vi "烧录座手动界面.vi"(8 "错误输入（无错误）":errorcluster, 10 "界面切换队列":refnum<queue>, 11 "VISA资源名称输入":refnum<visa-resource-name>) -> (0 "错误输出":errorcluster, 3 "VISA资源名称输出":refnum<visa-resource-name>)   [LabVIEW 2018]
panel:
  out "毫秒计时值":u32
  in  "枚举":T1(ring)
  in  "选项卡控件":enum32{"选项卡 1", "选项卡 2"}(tab)
  out "X30F":bool
  out "X30D":bool
  out "X30B":bool
  out "X309":bool
  out "X307":bool
  out "X305":bool
  out "X303":bool
  out "X301":bool
  out "X30E":bool
  out "X30C":bool
  out "X30A":bool
  out "X308":bool
  out "X306":bool
  out "X304":bool
  out "X302":bool
  out "写R747+读Y107+16#烧录启动":bool
  out "写R746+读Y106+14#烧录启动":bool
  out "写R745+读Y105+12#烧录启动":bool
  out "写R744+读Y104+10#烧录启动":bool
  out "写R743+读Y103+8#烧录启动":bool
  out "写R742+读Y102+6#烧录启动":bool
  out "写R741+读Y101+4#烧录启动":bool
  out "写R740+读Y100+2#烧录启动":bool
  out "写R9F+读Y30F+15#烧录启动":bool
  out "写R9E+读Y30E+13#烧录启动":bool
  out "写R9D+读Y30D+11#烧录启动":bool
  out "写R9C+读Y30C+9#烧录启动":bool
  out "写R9B+读Y30B+7#烧录启动":bool
  out "写R9A+读Y30A+5#烧录启动":bool
  out "写R99+读Y309+3#烧录启动":bool
  out "写R98+读Y308+1#烧录启动":bool
  out "写R7F+读Y307+8#烧录气缸":bool
  out "写R7E+读Y306+7#烧录气缸":bool
  out "写R7D+读Y305+6#烧录气缸":bool
  out "写R7C+读Y304+5#烧录气缸":bool
  out "写R7B+读Y303+4#烧录气缸":bool
  out "写R7A+读Y302+3#烧录气缸":bool
  out "写R79+读Y301+2#烧录气缸":bool
  out "写R78+读Y300+1#烧录气缸":bool
  out "DDT90356":dbl
  out "DDT90348":dbl
  out "自动界面":bool
  out "手动界面":bool
  out "参数界面":bool
  out "IO界面":bool
  out "产品界面":bool
  out "字符串":string
  out "DDT90352":dbl
  out "DDT90360":dbl
  out "通讯周期":dbl
  out "DT1184":T2(ring)
  out "写R0+读R1+手动启动":bool
  out "写R4+读R4+手动停止":bool
  out "写R8+读R9+机器复位":bool
  out "写R80+读R80+报警清除":bool
  out "手动5界面":bool
  out "X300":bool
  # "X"
  # "Z1"
  # "Z2"
  # "Y"
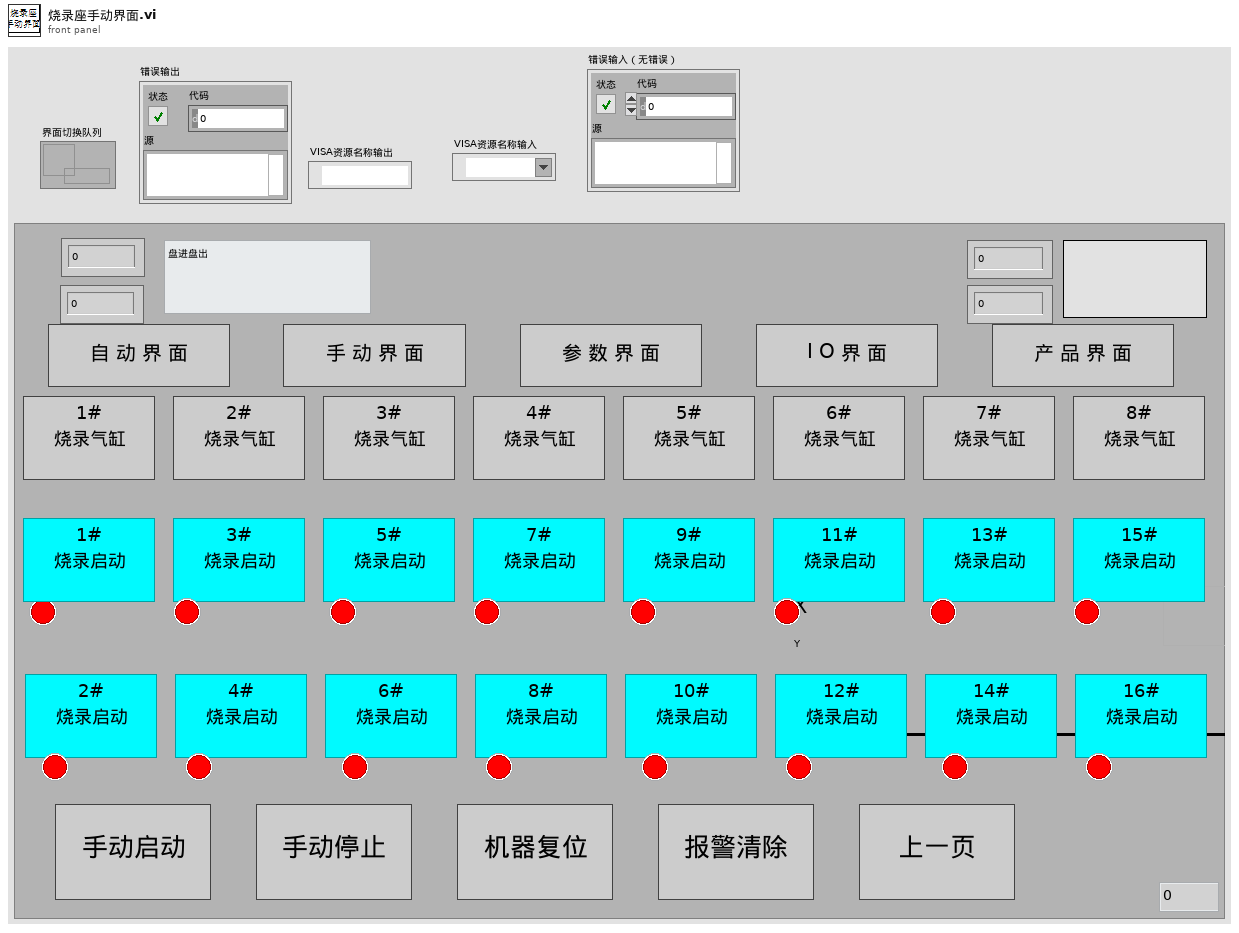
[diagram p1: front panel]
types:
  T1 = enum16{"读初始化", "读R80+8", "读R9+8", "读Y300+8", "读Y100+8", "读Y308+8", "读X308+8", "读X300+8", "读R1+8", "读DDT90356", "读DT1184", "读DDT90348", ""}
  T2 = enum16{"盘进盘出", "卷进卷出", "盘进卷出", "管进盘出", "管进卷出", "卷进盘出", ""}
  T3 = typedef "数据簇.ctl" = cluster{"字符串":string, "数值":i32, "布尔":bool}
  T4 = enum8{"Enabled", "Disabled", "Disabled and Grayed Out"}
  T5 = typedef "lveventtype.ctl" = enum32{"Null", "Timeout", "Annotation Menu Selection", "Annotation Menu Selection?", "App Instance Close", "App Instance Close?", "Autoscale Range Change", "Bookmark Info Change", "Cell Edit", "Cell Edit?", "Cursor Grab", "Cursor Grab?", "Cursor Menu Selection", "Cursor Menu Selection?", "Cursor Move", "Cursor Release", "Data Change", "Direction Change", "Display State Change", "Drag Ended", "Drag Enter", "Drag Leave", "Drag Over", "Drag Source Update", "Drag Starting", "Drag Starting?", "Drop", "Exec State Change", "Key Down", "Key Down?", "Key Repeat", "Key Repeat?", "Key Up", "Listbox Double Click", "Menu Activation?", "Menu Selection (App)", "Menu Selection? (App)", "Menu Selection (User)", "Mouse Down", "Mouse Down?", "Mouse Enter", "Mouse Leave", "Mouse Move", "Mouse Up", "Mouse Wheel", "NI Security User Change (App)", "Pane Size", "Panel Close", "Panel Close?", "Panel Resize", "Plot Attribute Change", "Scale Range Change", "Shortcut Menu Activation?", "Shortcut Menu Selection (App)", "Shortcut Menu Selection? (App)", "Shortcut Menu Selection (User)", "Tree Double Click", "Tree Drag", "Tree Drag?", "Tree Drop", "Tree Drop?", "Tree Item Close", "Tree Item Close?", "Tree Item Open", "Tree Item Open?", "User Event", "Value Change"}
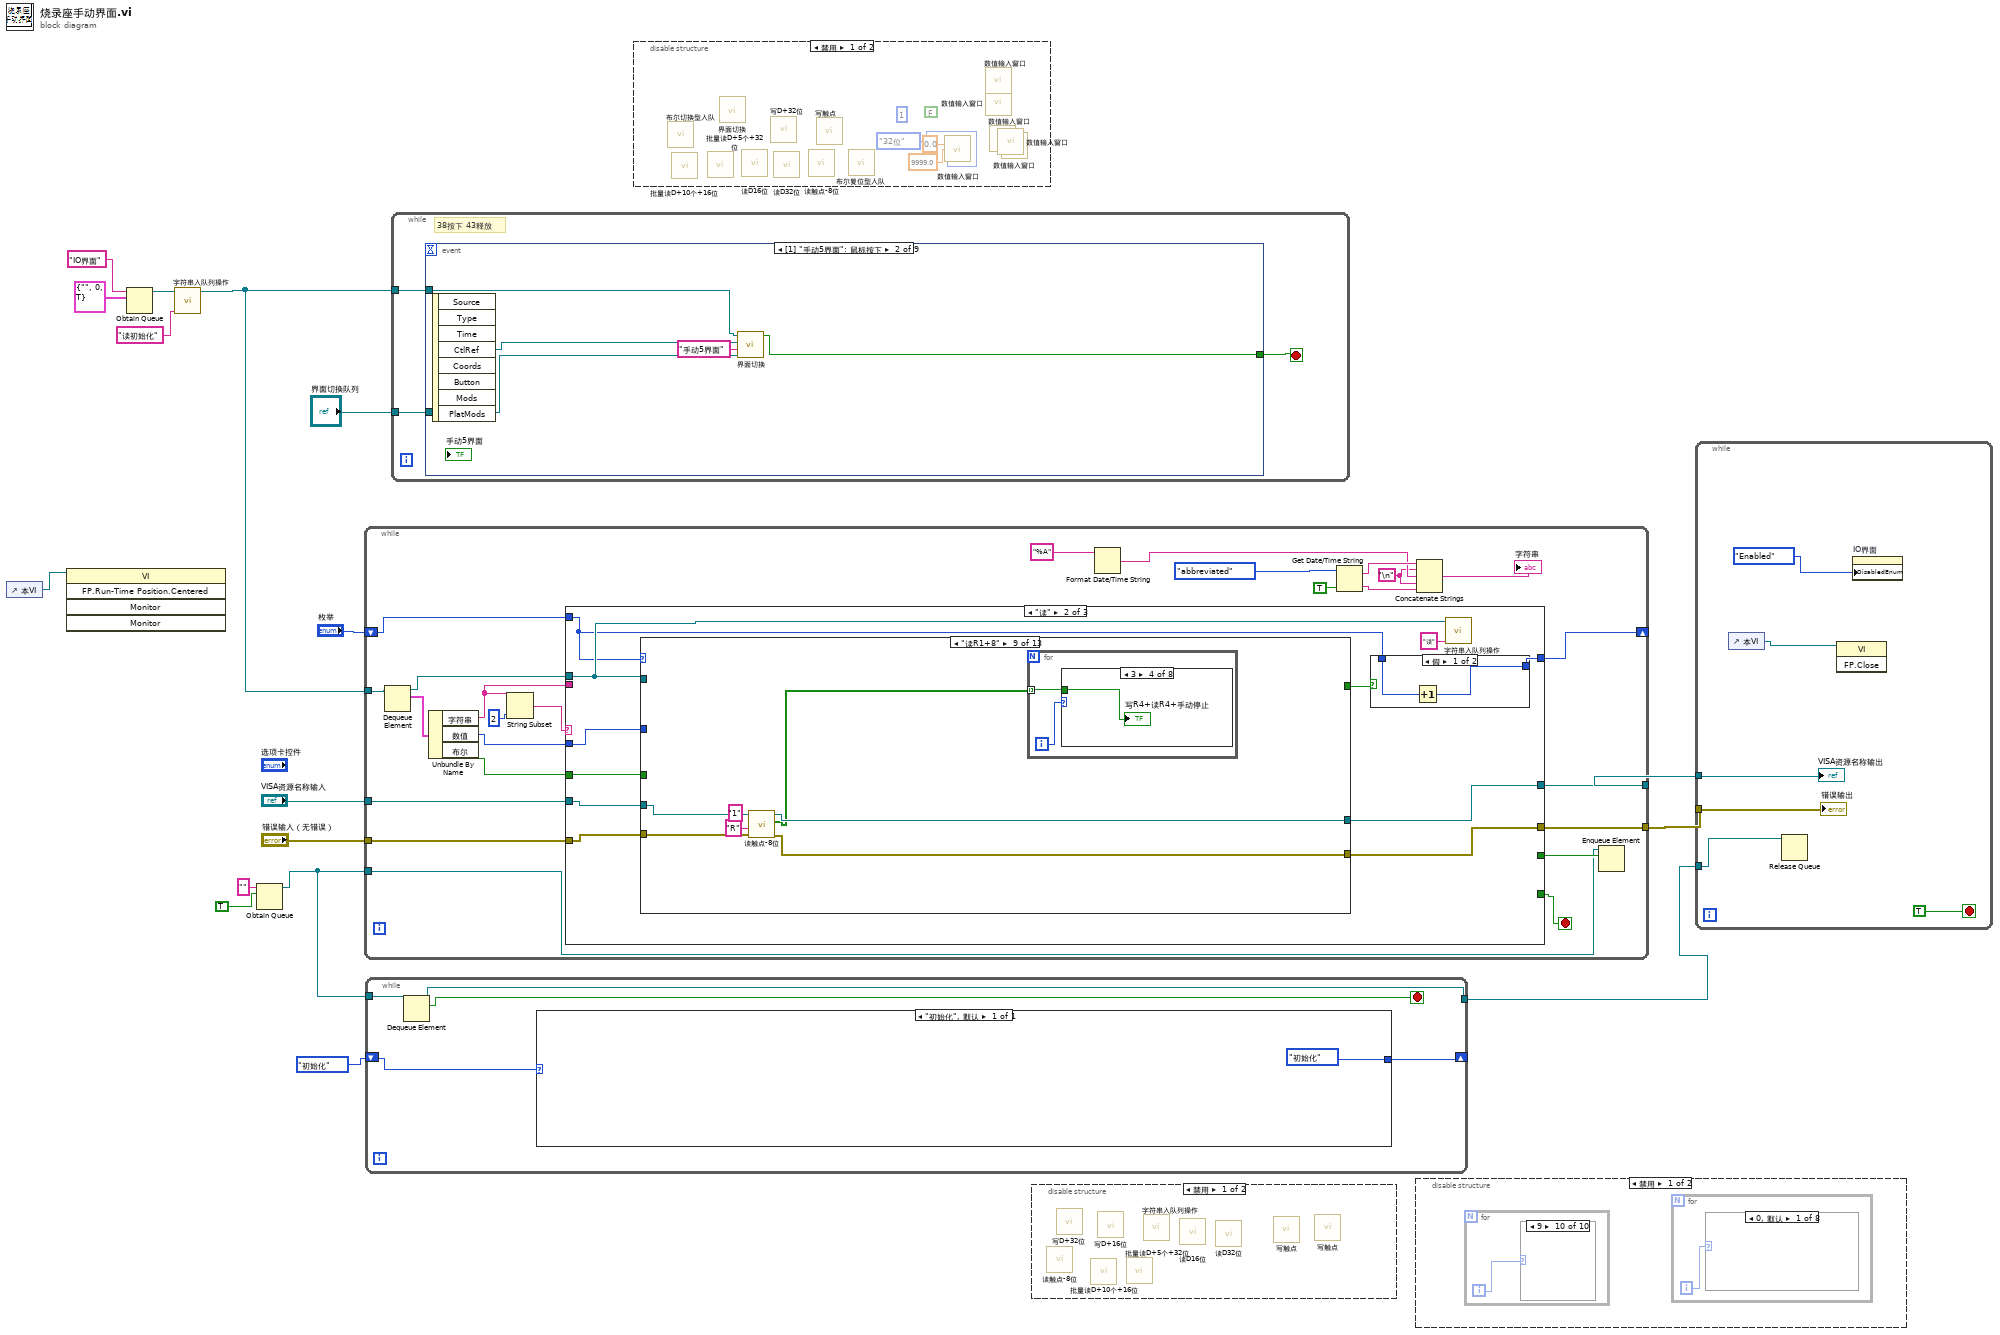
[diagram p0: block diagram]
diagram:
  n1 = control-ref of="本VI"() -> (w1:refnum<vi>)
  n2 = invoke class="VI" method="FP.Run-Time Position.Centered"(reference=w1) -> ()  [unwired: 4 in, 5 out]
  n3 = Obtain Queue(name (unnamed)="IO界面" ("名称（未命名）"), element data type=T3 {"字符串"="", "数值"=0, "布尔"=TRUE}) -> (queue out=w10:refnum<queue>)  [unwired: 3 in, 2 out]
  n4 = call "字符串入队列操作.vi"("字符消息入队列"="读初始化", "界面切换队列"=w10) -> ("队列输出"=w2:refnum<queue>)  [unwired: 9 in]
  n5 = Obtain Queue(name (unnamed)="" ("名称（未命名）"), element data type=TRUE) -> (queue out=w5:refnum<queue>)  [unwired: 3 in, 2 out]
  n6 = while {
    tunnel: w2 -> [w38]
    tunnel: "VISA资源名称输入" -> [w31]
    tunnel: "错误输入（无错误）" -> [w30]
    tunnel: [w29] -> w12
    tunnel: [w28] -> w11
    shift-right: [w25] -> _
    shift-left: "枚举" -> [w26]
    tunnel: w5 -> [w18]
    stop <- w20 stop-if-true
    w22 = "\n"
    n7 = Dequeue Element(queue=w38) -> (queue out=w35:refnum<queue>, element=w37:T3)  [unwired: 2 in, 2 out]
    n8 = Unbundle By Name(w37) -> ("字符串"=w32:string, "数值"=w34:i32, "布尔"=w33:bool)
    n9 = String Subset(string=w32, length (rest)=2 ("长度（剩余）")) -> (substring=w36:string)  [unwired: 1 in]
    n10 = case shown="\"读\"" w36 {
      selector: w36 -> [w45 _ _]
      tunnel: w35 -> [_ w53 w238]
      tunnel: w34 -> [_ w60 w237]
      tunnel: w33 -> [_ w59 w236]
      tunnel: w32 -> [_ _ w230]
      tunnel: w31 -> [w44 w58 w235]
      tunnel: w30 -> [w43 w57 w234]
      tunnel: [w44 w56 w232] -> w29
      tunnel: [w43 w55 w231] -> w28
      tunnel: [_ _ w233] -> w20
      tunnel: w26 -> [_ w51 _]
      tunnel: [_ w50 _] -> w25
      tunnel: [_ _ w228] -> w19
      frame "", Default {
        n11 = Concatenate Strings("无对应消息分支**" ("消息"), w45, "**" ("字符串"), "读写状态机" ("字符串")) -> (w47:string)
        n12 = One Button Dialog(message=w47) -> ()  [unwired: 1 in, 1 out]
      }
      frame "读" {
        n13 = case shown="\"读R1+8\"" w51 {
          tunnel: w53 -> [_ _ _ _ _ _ _ _ _ _ _ _ _]
          tunnel: w60 -> [_ _ _ _ _ _ _ _ _ _ _ _ _]
          tunnel: w58 -> [w65 w72 w82 w92 w109 w126 w143 w160 w177 w193 w202 w215 w227]
          tunnel: w57 -> [w64 w71 w81 w91 w108 w125 w142 w159 w176 w192 w201 w214 w226]
          tunnel: [w65 w68 w78 w88 w105 w122 w139 w156 w173 w191 w200 w213 w227] -> w56
          tunnel: [w64 w67 w77 w87 w104 w121 w138 w155 w172 w190 w199 w212 w226] -> w55
          tunnel: w59 -> [_ _ _ _ _ _ _ _ _ _ _ _ _]
          tunnel: [_ _ _ _ _ _ _ _ _ _ _ _ TRUE] -> w52
          frame "读初始化" {
            n14 = Tick Count (ms)() -> (millisecond timer value=→"毫秒计时值":u32)
          }
          frame "读R80+8" {
            n15 = call "读触点-8位.vi"("error out"=w71, "触点类型"="R", "读取起始地址"="80", "VISA resource name out"=w72) -> ("error IO"=w67:errorcluster, "读取布尔数组"=w66:bool[], "VISA resource name out 2"=w68:refnum<visa-resource-name>)  [unwired: 4 in, 1 out]
            n16 = for {
              tunnel: w66 -> [w73] mode=indexing
              i -> [w74]
              n17 = case shown="0, 默认" w74 {
                tunnel: w73 -> [w75 _ _ _ _ _ _ _]
                frame 0, Default {
                  "写R80+读R80+报警清除" <- w75
                }
                frame 1 {
                }
                frame 2 {
                }
                frame 3 {
                }
                frame 4 {
                }
                frame 5 {
                }
                frame 6 {
                }
                frame 7 {
                }
              }
            }
          }
          frame "读R9+8" {
            n18 = call "读触点-8位.vi"("error out"=w81, "触点类型"="R", "读取起始地址"="9", "VISA resource name out"=w82) -> ("error IO"=w77:errorcluster, "读取布尔数组"=w76:bool[], "VISA resource name out 2"=w78:refnum<visa-resource-name>)  [unwired: 4 in, 1 out]
            n19 = for {
              tunnel: w76 -> [w83] mode=indexing
              i -> [w84]
              n20 = case shown="0, 默认" w84 {
                tunnel: w83 -> [w85 _ _ _ _ _ _ _]
                frame 0, Default {
                  "写R8+读R9+机器复位" <- w85
                }
                frame 1 {
                }
                frame 2 {
                }
                frame 3 {
                }
                frame 4 {
                }
                frame 5 {
                }
                frame 6 {
                }
                frame 7 {
                }
              }
            }
          }
          frame "读Y300+8" {
            n21 = call "读触点-8位.vi"("error out"=w91, "触点类型"="Y", "读取起始地址"="300", "VISA resource name out"=w92) -> ("error IO"=w87:errorcluster, "读取布尔数组"=w86:bool[], "VISA resource name out 2"=w88:refnum<visa-resource-name>)  [unwired: 4 in, 1 out]
            n22 = for {
              tunnel: w86 -> [w93] mode=indexing
              i -> [w94]
              n23 = case shown="7" w94 {
                tunnel: w93 -> [w95 w96 w97 w98 w99 w100 w101 w102]
                frame 0, Default {
                  "写R78+读Y300+1#烧录气缸" <- w95
                }
                frame 1 {
                  "写R79+读Y301+2#烧录气缸" <- w96
                }
                frame 2 {
                  "写R7A+读Y302+3#烧录气缸" <- w97
                }
                frame 3 {
                  "写R7B+读Y303+4#烧录气缸" <- w98
                }
                frame 4 {
                  "写R7C+读Y304+5#烧录气缸" <- w99
                }
                frame 5 {
                  "写R7D+读Y305+6#烧录气缸" <- w100
                }
                frame 6 {
                  "写R7E+读Y306+7#烧录气缸" <- w101
                }
                frame 7 {
                  "写R7F+读Y307+8#烧录气缸" <- w102
                }
              }
            }
          }
          frame "读Y100+8" {
            n24 = call "读触点-8位.vi"("error out"=w108, "触点类型"="Y", "读取起始地址"="300", "VISA resource name out"=w109) -> ("error IO"=w104:errorcluster, "读取布尔数组"=w103:bool[], "VISA resource name out 2"=w105:refnum<visa-resource-name>)  [unwired: 4 in, 1 out]
            n25 = for {
              tunnel: w103 -> [w110] mode=indexing
              i -> [w111]
              n26 = case shown="7" w111 {
                tunnel: w110 -> [w112 w113 w114 w115 w116 w117 w118 w119]
                frame 0, Default {
                  "写R740+读Y100+2#烧录启动" <- w112
                }
                frame 1 {
                  "写R741+读Y101+4#烧录启动" <- w113
                }
                frame 2 {
                  "写R742+读Y102+6#烧录启动" <- w114
                }
                frame 3 {
                  "写R743+读Y103+8#烧录启动" <- w115
                }
                frame 4 {
                  "写R744+读Y104+10#烧录启动" <- w116
                }
                frame 5 {
                  "写R745+读Y105+12#烧录启动" <- w117
                }
                frame 6 {
                  "写R746+读Y106+14#烧录启动" <- w118
                }
                frame 7 {
                  "写R747+读Y107+16#烧录启动" <- w119
                }
              }
            }
          }
          frame "读Y308+8" {
            n27 = call "读触点-8位.vi"("error out"=w125, "触点类型"="Y", "读取起始地址"="300", "VISA resource name out"=w126) -> ("error IO"=w121:errorcluster, "读取布尔数组"=w120:bool[], "VISA resource name out 2"=w122:refnum<visa-resource-name>)  [unwired: 4 in, 1 out]
            n28 = for {
              tunnel: w120 -> [w127] mode=indexing
              i -> [w128]
              n29 = case shown="7" w128 {
                tunnel: w127 -> [w129 w130 w131 w132 w133 w134 w135 w136]
                frame 0, Default {
                  "写R98+读Y308+1#烧录启动" <- w129
                }
                frame 1 {
                  "写R99+读Y309+3#烧录启动" <- w130
                }
                frame 2 {
                  "写R9A+读Y30A+5#烧录启动" <- w131
                }
                frame 3 {
                  "写R9B+读Y30B+7#烧录启动" <- w132
                }
                frame 4 {
                  "写R9C+读Y30C+9#烧录启动" <- w133
                }
                frame 5 {
                  "写R9D+读Y30D+11#烧录启动" <- w134
                }
                frame 6 {
                  "写R9E+读Y30E+13#烧录启动" <- w135
                }
                frame 7 {
                  "写R9F+读Y30F+15#烧录启动" <- w136
                }
              }
            }
          }
          frame "读X308+8" {
            n30 = call "读触点-8位.vi"("error out"=w142, "触点类型"="X", "读取起始地址"="308", "VISA resource name out"=w143) -> ("error IO"=w138:errorcluster, "读取布尔数组"=w137:bool[], "VISA resource name out 2"=w139:refnum<visa-resource-name>)  [unwired: 4 in, 1 out]
            n31 = for {
              tunnel: w137 -> [w144] mode=indexing
              i -> [w145]
              n32 = case shown="7" w145 {
                tunnel: w144 -> [w146 w147 w148 w149 w150 w151 w152 w153]
                frame 0, Default {
                  "X308" <- w146
                }
                frame 1 {
                  "X309" <- w147
                }
                frame 2 {
                  "X30A" <- w148
                }
                frame 3 {
                  "X30B" <- w149
                }
                frame 4 {
                  "X30C" <- w150
                }
                frame 5 {
                  "X30D" <- w151
                }
                frame 6 {
                  "X30E" <- w152
                }
                frame 7 {
                  "X30F" <- w153
                }
              }
            }
          }
          frame "读X300+8" {
            n33 = call "读触点-8位.vi"("error out"=w159, "触点类型"="X", "读取起始地址"="300", "VISA resource name out"=w160) -> ("error IO"=w155:errorcluster, "读取布尔数组"=w154:bool[], "VISA resource name out 2"=w156:refnum<visa-resource-name>)  [unwired: 4 in, 1 out]
            n34 = for {
              tunnel: w154 -> [w161] mode=indexing
              i -> [w162]
              n35 = case shown="7" w162 {
                tunnel: w161 -> [w163 w164 w165 w166 w167 w168 w169 w170]
                frame 0, Default {
                  "X300" <- w163
                }
                frame 1 {
                  "X301" <- w164
                }
                frame 2 {
                  "X302" <- w165
                }
                frame 3 {
                  "X303" <- w166
                }
                frame 4 {
                  "X304" <- w167
                }
                frame 5 {
                  "X305" <- w168
                }
                frame 6 {
                  "X306" <- w169
                }
                frame 7 {
                  "X307" <- w170
                }
              }
            }
          }
          frame "读R1+8" {
            n36 = call "读触点-8位.vi"("error out"=w176, "触点类型"="R", "读取起始地址"="1", "VISA resource name out"=w177) -> ("error IO"=w172:errorcluster, "读取布尔数组"=w171:bool[], "VISA resource name out 2"=w173:refnum<visa-resource-name>)  [unwired: 4 in, 1 out]
            n37 = for {
              tunnel: w171 -> [w178] mode=indexing
              i -> [w179]
              n38 = case shown="3" w179 {
                tunnel: w178 -> [w180 _ _ w181 _ _ _ _]
                frame 0, Default {
                  "写R0+读R1+手动启动" <- w180
                }
                frame 1 {
                }
                frame 2 {
                }
                frame 3 {
                  "写R4+读R4+手动停止" <- w181
                }
                frame 4 {
                }
                frame 5 {
                }
                frame 6 {
                }
                frame 7 {
                }
              }
            }
          }
          frame "读DDT90356" {
            n39 = call "批量读D+5个+32位.vi"("error out"=w192, "读取D地址"=90356, "VISA resource name out"=w193) -> ("error IO"=w190:errorcluster, "数组"=w196:i32[], "VISA resource name out 2"=w191:refnum<visa-resource-name>)  [unwired: 5 in, 1 out]
            n40 = Index Array(array=w196, index #1=0 ("索引"), index #2=2 ("索引")) -> (element #1=w189:i32, element #2=w188:i32)
            n41 = To Double Precision Float(number=w189) -> (double precision float=w187:dbl)
            n42 = To Double Precision Float(number=w188) -> (double precision float=w184:dbl)
            n43 = Divide(x=w187, y=100.0) -> (x/y=→"DDT90356":dbl)
            n44 = Divide(x=w184, y=100.0) -> (x/y=→"DDT90360":dbl)
          }
          frame "读DT1184" {
            n45 = call "读D16位.vi"("error out"=w201, "读取D地址"=1184, "VISA resource name out"=w202) -> ("error IO"=w199:errorcluster, "数值"=→"DT1184":u32, "VISA resource name out 2"=w200:refnum<visa-resource-name>)  [unwired: 5 in, 1 out]
          }
          frame "读DDT90348" {
            n46 = call "批量读D+5个+32位.vi"("error out"=w214, "读取D地址"=90348, "VISA resource name out"=w215) -> ("error IO"=w212:errorcluster, "数组"=w219:i32[], "VISA resource name out 2"=w213:refnum<visa-resource-name>)  [unwired: 5 in, 1 out]
            n47 = Index Array(array=w219, index #1=0 ("索引"), index #2=2 ("索引")) -> (element #1=w211:i32, element #2=w210:i32)
            n48 = To Double Precision Float(number=w210) -> (double precision float=w205:dbl)
            n49 = To Double Precision Float(number=w211) -> (double precision float=w209:dbl)
            n50 = Divide(x=w205, y=100.0) -> (x/y=→"DDT90352":dbl)
            n51 = Divide(x=w209, y=100.0) -> (x/y=→"DDT90348":dbl)
          }
          frame "" {
            n52 = local read "毫秒计时值"() -> (w223:u32)
            n53 = Tick Count (ms)() -> (millisecond timer value=w224:u32)
            n54 = Subtract(x=w224, y=w223) -> (x-y=w222:u32)
            n55 = Divide(x=w222, y=u32 1000) -> (x/y=→"通讯周期":dbl)
          }
        }
        n56 = case shown="假" w52 {
          tunnel: w51 -> [w62 _]
          tunnel: [w61 _] -> w50
          frame False {
            n57 = Increment(x=w62) -> (x+1=w61:T1)
          }
          frame True {
          }
        }
        n58 = call "字符串入队列操作.vi"("字符消息入队列"="读", "界面切换队列"=w53) -> ()  [unwired: 9 in, 1 out]
      }
      frame "写" {
        n59 = call "状态匹配.vi"("输入状态"=w230) -> ("输出状态"=w229:string)  [unwired: 10 in]
        n60 = case shown="\"写退出\"" w229 {
          selector: w229 -> [w241 _ _ _ _]
          tunnel: w238 -> [_ _ _ _ w281]
          tunnel: w237 -> [_ w247 w264 _ _]
          tunnel: w236 -> [_ _ _ w275 _]
          tunnel: w235 -> [w240 w257 w268 w280 w286]
          tunnel: w234 -> [w239 w256 w267 w279 w285]
          tunnel: [_ _ _ _ w284] -> w233
          tunnel: [w240 w255 w266 w278 w286] -> w232
          tunnel: [w239 w254 w265 w277 w285] -> w231
          tunnel: w230 -> [_ w246 w258 w269 _]
          tunnel: [_ _ _ _ w284] -> w228
          frame "", Default {
            n61 = Concatenate Strings("无对应消息分支**" ("消息"), w241, "**" ("字符串"), "写状态机" ("字符串")) -> (w245:string)
            n62 = One Button Dialog(message=w245) -> ()  [unwired: 1 in, 1 out]
          }
          frame "写DT" {
            n63 = String Length(string=w246) -> (length=w252:i32)
            n64 = Subtract(x=w252, y=4) -> (x-y=w250:i32)
            n65 = String Subset(string=w246, offset (0)=4 ("偏移量(0)"), length (rest)=w250) -> (substring=w249:string)
            n66 = Decimal String To Number(string=w249) -> (number=w248:i32)  [unwired: 2 in, 1 out]
            n67 = call "写D+16位.vi"("error out"=w256, "输入数值"=w247, "输入地址D"=w248, "VISA resource name out"=w257) -> ("error out 2"=w254:errorcluster, "VISA resource name out 2"=w255:refnum<visa-resource-name>)  [unwired: 3 in, 3 out]
          }
          frame "写DDT" {
            n68 = String Length(string=w258) -> (length=w262:i32)
            n69 = Subtract(x=w262, y=5) -> ()  [unwired: 1 out]
            n70 = String Subset(string=w258, offset (0)=5 ("偏移量(0)")) -> (substring=w259:string)  [unwired: 1 in]
            n71 = Decimal String To Number(string=w259) -> (number=w260:i32)  [unwired: 2 in, 1 out]
            n72 = call "写D+32位.vi"("error out"=w267, "输入数值"=w264, "输入地址D"=w260, "VISA resource name out"=w268) -> ("error out 2"=w265:errorcluster, "VISA resource name out 2"=w266:refnum<visa-resource-name>)  [unwired: 4 in, 2 out]
          }
          frame "写R" {
            n73 = String Length(string=w269) -> (length=w273:i32)
            n74 = Subtract(x=w273, y=3) -> (x-y=w271:i32)
            n75 = String Subset(string=w269, offset (0)=3 ("偏移量(0)"), length (rest)=w271) -> (substring=w270:string)
            n76 = call "写触点.vi"("布尔"=w275, "error out"=w279, "触点类型"="R", "写入起始地址"=w270, "VISA resource name out"=w280) -> ("error IO"=w277:errorcluster, "VISA resource name out 2"=w278:refnum<visa-resource-name>)  [unwired: 4 in, 1 out]
          }
          frame "写退出" {
            w284 = TRUE
            n77 = Flush Queue(queue=w281) -> (queue out=w282:refnum<queue>, error out=w283:errorcluster)  [unwired: 1 in, 1 out]
            n78 = Release Queue(queue=w282, error in (no error)=w283) -> ()  [unwired: 1 in, 3 out]
          }
        }
      }
    }
    n79 = Format Date/Time String(time format string (%c)="%A" ("时间格式字符串(%c)")) -> (date/time string=w23:string)  [unwired: 2 in]
    n80 = Get Date/Time String(date format (0)=enum16{"short", "long", "abbreviated"}."abbreviated" ("日期格式(0)"), want seconds? (F)=TRUE ("需要秒？(F)")) -> (date string=w40:string, time string=w21:string)  [unwired: 1 in]
    n81 = Concatenate Strings(w40, w22, w23, w22, w21) -> (→"字符串":string)
    n82 = Enqueue Element(queue=w18, element=w19) -> ()  [unwired: 2 in, 3 out]
  }
  n83 = while {
    shift-right: [w290] -> _
    shift-left: enum16{"初始化"}."初始化" -> [w291]
    tunnel: w5 -> [w289]
    tunnel: [w287] -> w4
    stop <- w288 stop-if-true
    n84 = Dequeue Element(queue=w289) -> (queue out=w287:refnum<queue>, element=w288:bool)  [unwired: 2 in, 2 out]
    n85 = case shown="\"初始化\", 默认" w291 {
      tunnel: [enum16{"初始化"}."初始化"] -> w290
      frame "初始化", Default {
      }
    }
  }
  n86 = while {
    tunnel: w2 -> [w294]
    tunnel: "界面切换队列" -> [w293]
    stop <- w295 stop-if-true
    # "38按下 43释放"
    n87 = event shown="[1] \"手动5界面\": 鼠标按下" {
      selector: _ -> [_ _ _ _ _ _ _ _ _]
      dyn-events: _ -> [_ _ _ _ _ _ _ _ _]
      timeout: _ -> [_ _ _ _ _ _ _ _ _]
      tunnel: [TRUE w308 _ w317 w322 w327 w332 _ w339] -> w295
      tunnel: w294 -> [w298 w309 w316 w321 w326 w331 w336 _ w338]
      tunnel: w293 -> [w297 w307 _ w320 w325 w330 w335 _ w337]
      event "IO界面": Mouse Down {
        n88 = event-data() -> ("CtlRef"=w300:refnum<vi>)  [unwired: 1 in, 7 out]
        n89 = property class="Bool"(reference=w300) -> ("DisabledEnum"=w299:T4)  [unwired: 1 in, 2 out]
        n90 = case shown="\"Enabled\", 默认" w299 {
          tunnel: w298 -> [w302 _]
          tunnel: w297 -> [w303 _]
          frame "Enabled", Default {
            n91 = call "字符串入队列操作.vi"("字符消息入队列"="写退出", "界面切换队列"=w302) -> ()  [unwired: 9 in, 1 out]
            n92 = call "字符串入队列操作.vi"("字符消息入队列"="IO界面" ("界面切换消息入队列"), "界面切换队列"=w303) -> ()  [unwired: 9 in, 1 out]
          }
          frame "Disabled" {
          }
        }
      }
      event "手动5界面": Mouse Down {
        n93 = event-data() -> ("CtlRef"=w306:refnum<vi>)  [unwired: 1 in, 7 out]
        n94 = call "界面切换.vi"("界面切换队列输入"=w307, "切换界面名称输入"="手动5界面", "Bool引用句柄"=w306, "状态转移输入"=w309) -> ("布尔"=w308:bool)  [unwired: 7 in]
      }
      event "写R0+读R1+手动启动", "写R4+读R4+手动停止", "写R8+读R9+机器复位", "写R80+读R80+报警清除", "写R78+读Y300+1#烧录气缸", "写R79+读Y301+2#烧录气缸", "写R7A+读Y302+3#烧录气缸", "写R7B+读Y303+4#烧录气缸", "写R7C+读Y304+5#烧录气缸", "写R7D+读Y305+6#烧录气缸", "写R7E+读Y306+7#烧录气缸", "写R98+读Y308+1#烧录启动", "写R99+读Y309+3#烧录启动", "写R9A+读Y30A+5#烧录启动", "写R9B+读Y30B+7#烧录启动", "写R9C+读Y30C+9#烧录启动", "写R9D+读Y30D+11#烧录启动", "写R9E+读Y30E+13#烧录启动", "写R9F+读Y30F+15#烧录启动", "写R740+读Y100+2#烧录启动", "写R741+读Y101+4#烧录启动", "写R742+读Y102+6#烧录启动", "写R743+读Y103+8#烧录启动", "写R744+读Y104+10#烧录启动", "写R745+读Y105+12#烧录启动", "写R746+读Y106+14#烧录启动", "写R747+读Y107+16#烧录启动": Mouse Down; "写R0+读R1+手动启动", "写R4+读R4+手动停止", "写R8+读R9+机器复位", "写R78+读Y300+1#烧录气缸", "写R79+读Y301+2#烧录气缸", "写R7A+读Y302+3#烧录气缸", "写R7B+读Y303+4#烧录气缸", "写R7C+读Y304+5#烧录气缸", "写R7D+读Y305+6#烧录气缸", "写R7E+读Y306+7#烧录气缸", "写R98+读Y308+1#烧录启动", "写R99+读Y309+3#烧录启动", "写R9A+读Y30A+5#烧录启动", "写R9B+读Y30B+7#烧录启动", "写R9C+读Y30C+9#烧录启动", "写R9D+读Y30D+11#烧录启动", "写R9E+读Y30E+13#烧录启动", "写R9F+读Y30F+15#烧录启动", "写R740+读Y100+2#烧录启动", "写R741+读Y101+4#烧录启动", "写R742+读Y102+6#烧录启动", "写R743+读Y103+8#烧录启动", "写R744+读Y104+10#烧录启动", "写R745+读Y105+12#烧录启动", "写R746+读Y106+14#烧录启动", "写R747+读Y107+16#烧录启动", "写R80+读R80+报警清除": Mouse Up {
        n95 = event-data() -> ("Type"=w315:T5, "CtlRef"=w314:refnum<vi>)  [unwired: 1 in, 6 out]
        n96 = property class="Bool"(reference=w314) -> (reference out=w313:refnum<vi>, "Label.Text"=w312:string)  [unwired: 1 in, 1 out]
        n97 = Match Pattern(string=w312, regular expression="+" ("正则表达式")) -> (before substring=w310:string)  [unwired: 1 in, 3 out]
        n98 = call "布尔复位型入队.vi"("队列输入"=w316, "数值"=w315, "控件引用"=w313, "字符消息入队列"=w310) -> ()  [unwired: 2 in, 3 out]
      }
      event "参数界面": Mouse Down {
        n99 = event-data() -> ("CtlRef"=w319:refnum<vi>)  [unwired: 1 in, 7 out]
        n100 = call "界面切换.vi"("界面切换队列输入"=w320, "切换界面名称输入"="参数界面", "Bool引用句柄"=w319, "状态转移输入"=w321) -> ("布尔"=w317:bool)  [unwired: 7 in]
      }
      event "产品界面": Mouse Down {
        n101 = event-data() -> ("CtlRef"=w324:refnum<vi>)  [unwired: 1 in, 7 out]
        n102 = call "界面切换.vi"("界面切换队列输入"=w325, "切换界面名称输入"="产品界面", "Bool引用句柄"=w324, "状态转移输入"=w326) -> ("布尔"=w322:bool)  [unwired: 7 in]
      }
      event "手动界面": Mouse Down {
        n103 = event-data() -> ("CtlRef"=w329:refnum<vi>)  [unwired: 1 in, 7 out]
        n104 = call "界面切换.vi"("界面切换队列输入"=w330, "切换界面名称输入"="手动界面", "Bool引用句柄"=w329, "状态转移输入"=w331) -> ("布尔"=w327:bool)  [unwired: 7 in]
      }
      event "自动界面": Mouse Down {
        n105 = event-data() -> ("CtlRef"=w334:refnum<vi>)  [unwired: 1 in, 7 out]
        n106 = call "界面切换.vi"("界面切换队列输入"=w335, "切换界面名称输入"="自动界面", "Bool引用句柄"=w334, "状态转移输入"=w336) -> ("布尔"=w332:bool)  [unwired: 7 in]
      }
      event Timeout {
        n107 = event-data() -> ()  [unwired: 1 in, 3 out]
      }
      event Panel Close? {
        n108 = event-data() -> ()  [unwired: 1 in, 4 out]
        n109 = Two Button Dialog(message="确定退出程序？" ("消息")) -> (T button?=w340:bool)  [unwired: 2 in]
        n110 = case shown="假" w340 {
          tunnel: [_ TRUE] -> w339
          tunnel: w338 -> [_ w345]
          tunnel: w337 -> [_ w344]
          frame False {
          }
          frame True {
            n111 = call "字符串入队列操作.vi"("字符消息入队列"="退出", "界面切换队列"=w344) -> ()  [unwired: 9 in, 1 out]
            n112 = call "字符串入队列操作.vi"("字符消息入队列"="写退出", "界面切换队列"=w345) -> ()  [unwired: 9 in, 1 out]
          }
        }
        n113 = event-data("Discard?"=TRUE ("放弃？")) -> ()  [unwired: 1 in, 1 out]
      }
    }
  }
  n114 = disable-structure shown="禁用" {
    frame Disabled {
      (unwired) u32 1 ("转换比例")
      (unwired) FALSE ("忽略数值上下限")
      n115 = call "布尔切换型入队.vi"() -> ()  [unwired: 12 in]
      n116 = call "批量读D+10个+16位.vi"() -> ()  [unwired: 8 in, 4 out]
      n117 = call "批量读D+5个+32位.vi"() -> ()  [unwired: 8 in, 4 out]
      n118 = call "界面切换.vi"() -> ()  [unwired: 11 in, 1 out]
      n119 = call "读D16位.vi"() -> ()  [unwired: 8 in, 4 out]
      n120 = call "写D+32位.vi"() -> ()  [unwired: 8 in, 4 out]
      n121 = call "读D32位.vi"() -> ()  [unwired: 9 in, 3 out]
      n122 = call "读触点-8位.vi"() -> ()  [unwired: 8 in, 4 out]
      n123 = call "写触点.vi"() -> ()  [unwired: 9 in, 3 out]
      n124 = call "布尔复位型入队.vi"() -> ()  [unwired: 6 in, 3 out]
      n125 = call "数值输入窗口.vi"("输入下限"=0.0, "输入上限"=9999.0, "数据类型"=enum16{"32位", "16位"}."32位") -> ("转换比例"=w351:u32)  [unwired: 9 in, 3 out]
      n126 = call "数值输入窗口.vi"() -> ()  [unwired: 13 in, 3 out]
      n127 = call "数值输入窗口.vi"() -> ()  [unwired: 13 in, 3 out]
      n128 = call "数值输入窗口.vi"() -> ()  [unwired: 13 in, 3 out]
      n129 = call "数值输入窗口.vi"() -> ()  [unwired: 13 in, 3 out]
      n130 = call "数值输入窗口.vi"() -> ()  [unwired: 13 in, 3 out]
    }
    frame Enabled {
    }
  }
  n131 = disable-structure shown="禁用" {
    frame Disabled {
      n132 = call "读触点-8位.vi"() -> ()  [unwired: 8 in, 4 out]
      n133 = call "写D+32位.vi"() -> ()  [unwired: 8 in, 4 out]
      n134 = call "批量读D+10个+16位.vi"() -> ()  [unwired: 8 in, 4 out]
      n135 = call "写D+16位.vi"() -> ()  [unwired: 7 in, 5 out]
      n136 = call "批量读D+5个+32位.vi"() -> ()  [unwired: 8 in, 4 out]
      n137 = call "字符串入队列操作.vi"() -> ()  [unwired: 11 in, 1 out]
      n138 = call "读D16位.vi"() -> ()  [unwired: 8 in, 4 out]
      n139 = call "读D32位.vi"() -> ()  [unwired: 9 in, 3 out]
      n140 = call "写触点.vi"() -> ()  [unwired: 9 in, 3 out]
      n141 = call "写触点.vi"() -> ()  [unwired: 9 in, 3 out]
    }
    frame Enabled {
    }
  }
  n142 = disable-structure shown="禁用" {
    frame Disabled {
      n143 = for {
        i -> [w353]
        n144 = case shown="9" w353 {
          frame 0, Default {
          }
          frame 1 {
          }
          frame 2 {
          }
          frame 3 {
          }
          frame 4 {
          }
          frame 5 {
          }
          frame 6 {
          }
          frame 7 {
          }
          frame 8 {
          }
          frame 9 {
          }
        }
      }
      n145 = for {
        i -> [w352]
        n146 = case shown="0, 默认" w352 {
          frame 0, Default {
          }
          frame 1 {
          }
          frame 2 {
          }
          frame 3 {
          }
          frame 4 {
          }
          frame 5 {
          }
          frame 6 {
          }
          frame 7 {
          }
        }
      }
    }
    frame Enabled {
    }
  }
  n147 = while {
    tunnel: w12 -> [w358]
    tunnel: w11 -> [w357]
    tunnel: w4 -> [w356]
    stop <- TRUE stop-if-true
    n148 = control-ref of="本VI"() -> (w354:refnum<vi>)
    n149 = Release Queue(queue=w356) -> ()  [unwired: 2 in, 3 out]
    n150 = invoke class="VI" method="FP.Close"(reference=w354) -> ()  [unwired: 2 in, 3 out]
    n151 = property on="IO界面" class="Bool"("DisabledEnum"=T4."Enabled" ("禁用")) -> ()  [unwired: 2 in, 2 out]
    "VISA资源名称输出" <- w358
    "错误输出" <- w357
  }
